vi "LUCS001RT_Navigation1_DataExchanger.vi"(7 "GPS DataIn":T1={"WayPointDataGood"=TRUE, "Waypoint:XTE"=0.01, "Waypoint:SteeringDirection"="L", "WayPoint:OriginID"="", "Waypoint:DestinationID"="", "DestinationWaypoint.Latitude.Deg"=0, "DestinationWaypoint.Latitude.Min"=0.0, "DestinationWaypointLatitude.North/South"="", "DestinationWaypointLongitude.Deg"=0, "DestinationWaypointLongitude.Min"=0.0, "DestinationWaypointLongitude.East/West"="", "RangeToDestination(NauticalMiles)"=0.0, "TrueBearingToDestination"=33.7, "VelocityTowardsDestination(Knots)"=0.0, "ArrivalAlarm"=TRUE, "ITOW"=247, "TAcc"=0, "LON"=0.0, "LAT"=0.0, "HEIGHT"=0, "HMSL"=0, "Hacc"=0, "Vacc"=0, "MSTOW"=0, "FixType"=0, "ECEF_X_Coor"=0, "ECEF_Y_Coor"=0, "ECEF_Z_Coor"=0, "Pacc"=0, "ECEF_X_Vlsty"=0, "ECEF_Y_Vlsty"=0, "ECEF_Z_Vlsty"=0, "Sacc"=0, "PosDOP"=0, "#SatsInNavSol"=0, "NED_NVsty"=0, "NED_Evsty"=0, "NED_DNvsty"=0, "Speed(3-D)"=0, "GSpeed(2-D)"=0, "Heading(2-D)"=0.0, "CAcc"=0, "Nano"=0, "Year"=0, "Month"=0, "Day"=0, "Hour"=0, "Min"=0, "Sec"=0, "UTC Valid"=0} {"UTC Valid" items=["UTC not valid", "Valid Time of Week", "Valid Week Number", "NA", "Valid UTC"]; "CAcc" format="%.0f°"; "Heading(2-D)" format="%0.6f°"; "GSpeed(2-D)" format="%.0f cm/s"; "Speed(3-D)" format="%.0f cm/s"; "NED_DNvsty" format="%.0f cm/s"; "NED_Evsty" format="%.0f cm/s"; "NED_NVsty" format="%.0f cm/s"; "Sacc" format="%.0f cm/s"; "ECEF_Z_Vlsty" format="%.0f cm/s"; "ECEF_Y_Vlsty" format="%.0f cm/s"; "ECEF_X_Vlsty" format="%.0f cm/s"; "FixType" items=["No Fix", "Dead Reckoning Only", "2D-Fix", "3D-Fix", "GPS + Dead Reckoning", "Time Only Fix", "RESERVED"]; "Vacc" format="%.0f mm"; "Hacc" format="%.0f mm"; "HMSL" format="%d mm"; "HEIGHT" format="%.0f mm"; "LAT" format="%#.6f"; "LON" format="%#.6f"; "Waypoint:XTE" format="%#.2f"}, 8 "error in (no error)":errorcluster, 11 "NavParam":T3={"Lat1Hem"=33.0, "Lat1Rad"=57.0, "Lon1Hem"=0.0, "Lon1Rad"=0.0, "Lat2Hem"=118.0, "Lat2Rad"=24.0, "Lon2Hem"=0.0, "Lon2Rad"=0.0, "DistanceRad"=40.0, "DistanceNM"=38.0, "CourseCond"=0.0, "TrueCourseRad"=0.0, "LatDegCurr"=73, "LatMinCurr"=47.0, "LatHemCurr"=0.0, "LatRadCurr"=0.0, "LonDegCurr"=0, "LonMinCurr"=0.0, "LonHemCurr"=0.0, "LonRadCurr"=-0.7023601432666094, "XTD"=40.0, "DistCurrRad"=38.0, "TrueCourseCurrRad"=0.0, "DistCurrNM"=0.7091854527270293, "TrueCourseDeg"=73.0, "TrueCourseCurrDeg"=47.0, "LON1"=0.0, "LAT1"=1.2877620997631494, "LON2"=38.0, "LAT2"=38.0} {"DistanceNM" format="%#.3f"}) -> (0 "error out":errorcluster, 3 "NavParamOut":T2={"Lat1Hem"=33.0, "Lat1Rad"=57.0, "Lon1Hem"=0.0, "Lon1Rad"=0.5925392810520749, "Lat2Hem"=118.0, "Lat2Rad"=24.0, "Lon2Hem"=0.0, "Lon2Rad"=2.066469834361286, "DistanceRad"=40.0, "DistanceNM"=38.0, "CourseCond"=0.0, "TrueCourseRad"=0.7091854527270293, "LatDegCurr"=73, "LatMinCurr"=47.0, "LatHemCurr"=0.0, "LatRadCurr"=1.2877620997631494, "LonDegCurr"=1, "LonMinCurr"=2143.726101388629, "LonHemCurr"=-0.7023601432666094, "LonRadCurr"=-0.7023601432666094, "XTD"=40.0, "DistCurrRad"=38.0, "TrueCourseCurrRad"=0.0, "DistCurrNM"=0.7091854527270293, "TrueCourseDeg"=73.0, "TrueCourseCurrDeg"=47.0, "LON1"=0.0, "LAT1"=1.2877620997631494, "LON2"=38.0, "LAT2"=38.0} {"DistanceNM" format="%#.3f"})   [LabVIEW 2020]
uses:
  TypeDefs/NavigationParams.ctl
  LUCS001RT_GPS_Data.ctl
  GPS_Navigation_Parameters.ctl
panel:
  # "WAYPOINT"
  # "CURRENT POSITION"
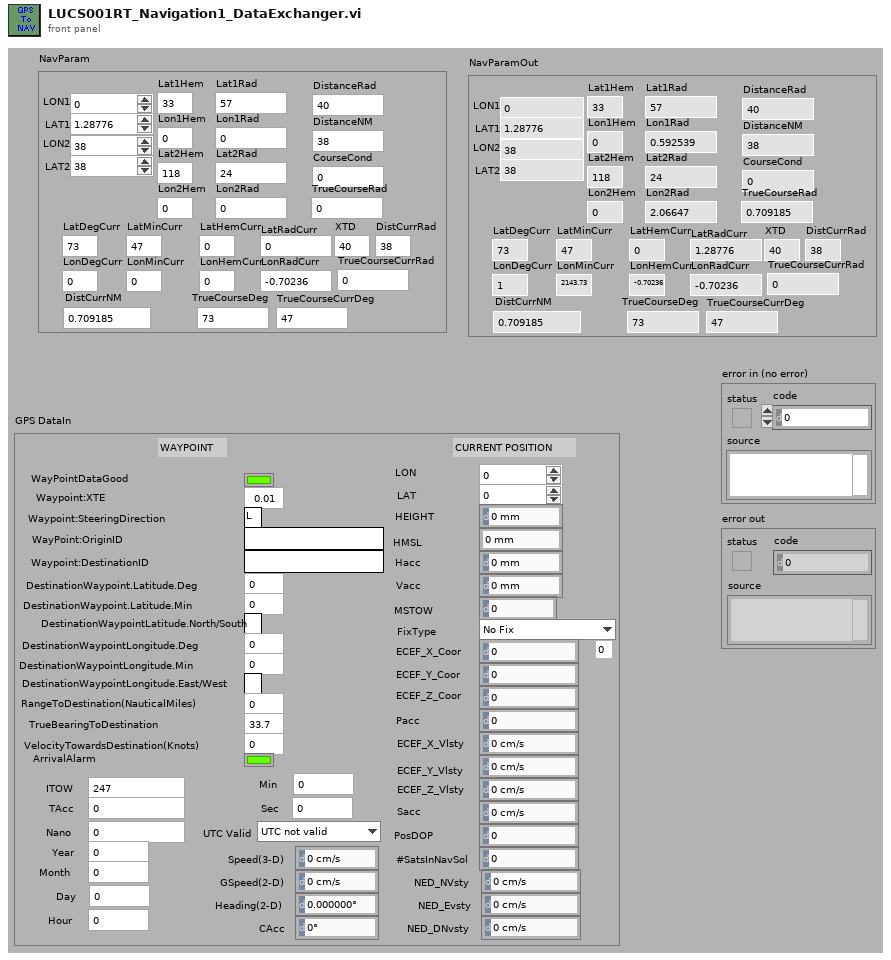
[diagram p1: front panel]
types:
  T1 = typedef "LUCS001RT_GPS_Data.ctl" = cluster{"WayPointDataGood":bool, "Waypoint:XTE":dbl, "Waypoint:SteeringDirection":string, "WayPoint:OriginID":string, "Waypoint:DestinationID":string, "DestinationWaypoint.Latitude.Deg":i32, "DestinationWaypoint.Latitude.Min":dbl, "DestinationWaypointLatitude.North/South":string, "DestinationWaypointLongitude.Deg":i32, "DestinationWaypointLongitude.Min":dbl, "DestinationWaypointLongitude.East/West":string, "RangeToDestination(NauticalMiles)":dbl, "TrueBearingToDestination":dbl, "VelocityTowardsDestination(Knots)":dbl, "ArrivalAlarm":bool, "ITOW":u32, "TAcc":u32, "LON":dbl, "LAT":dbl, "HEIGHT":i32, "HMSL":i32, "Hacc":u32, "Vacc":u32, "MSTOW":u32, "FixType":u8, "ECEF_X_Coor":i32, "ECEF_Y_Coor":i32, "ECEF_Z_Coor":i32, "Pacc":u32, "ECEF_X_Vlsty":i32, "ECEF_Y_Vlsty":i32, "ECEF_Z_Vlsty":i32, "Sacc":u32, "PosDOP":u16, "#SatsInNavSol":u8, "NED_NVsty":i32, "NED_Evsty":i32, "NED_DNvsty":i32, "Speed(3-D)":u32, "GSpeed(2-D)":u32, "Heading(2-D)":dbl, "CAcc":u32, "Nano":i32, "Year":u16, "Month":u8, "Day":u8, "Hour":u8, "Min":u8, "Sec":u8, "UTC Valid":u8}
  T2 = typedef "NavigationParams.ctl" = cluster{"Lat1Hem":dbl, "Lat1Rad":dbl, "Lon1Hem":dbl, "Lon1Rad":dbl, "Lat2Hem":dbl, "Lat2Rad":dbl, "Lon2Hem":dbl, "Lon2Rad":dbl, "DistanceRad":dbl, "DistanceNM":dbl, "CourseCond":dbl, "TrueCourseRad":dbl, "LatDegCurr":i32, "LatMinCurr":dbl, "LatHemCurr":dbl, "LatRadCurr":dbl, "LonDegCurr":i32, "LonMinCurr":dbl, "LonHemCurr":dbl, "LonRadCurr":dbl, "XTD":dbl, "DistCurrRad":dbl, "TrueCourseCurrRad":dbl, "DistCurrNM":dbl, "TrueCourseDeg":dbl, "TrueCourseCurrDeg":dbl, "LON1":dbl, "LAT1":dbl, "LON2":dbl, "LAT2":dbl}
  T3 = typedef "GPS_Navigation_Parameters.ctl" = cluster{"Lat1Hem":dbl, "Lat1Rad":dbl, "Lon1Hem":dbl, "Lon1Rad":dbl, "Lat2Hem":dbl, "Lat2Rad":dbl, "Lon2Hem":dbl, "Lon2Rad":dbl, "DistanceRad":dbl, "DistanceNM":dbl, "CourseCond":dbl, "TrueCourseRad":dbl, "LatDegCurr":i32, "LatMinCurr":dbl, "LatHemCurr":dbl, "LatRadCurr":dbl, "LonDegCurr":i32, "LonMinCurr":dbl, "LonHemCurr":dbl, "LonRadCurr":dbl, "XTD":dbl, "DistCurrRad":dbl, "TrueCourseCurrRad":dbl, "DistCurrNM":dbl, "TrueCourseDeg":dbl, "TrueCourseCurrDeg":dbl, "LON1":dbl, "LAT1":dbl, "LON2":dbl, "LAT2":dbl}
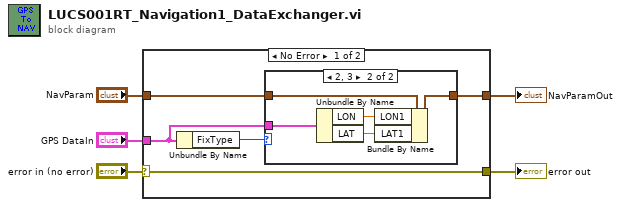
[diagram p0: block diagram]
diagram:
  n1 = case shown="No Error" "error in (no error)" {
    selector: "error in (no error)" -> [w10 w17]
    tunnel: "NavParam" -> [w7 _]
    tunnel: [w10 w17] -> w3
    tunnel: "GPS DataIn" -> [w8 _]
    tunnel: [w6 _] -> w1
    frame No Error {
      n2 = Unbundle By Name(w8) -> ("FixType"=w9:u8)
      n3 = case shown="2, 3" w9 {
        tunnel: w8 -> [_ w16]
        tunnel: w7 -> [w11 w15]
        tunnel: [w11 w12] -> w6
        frame 0, Default {
        }
        frame 2, 3 {
          n4 = Unbundle By Name(w16) -> ("LON"=w14:dbl, "LAT"=w13:dbl)
          n5 = Bundle By Name(cluster=w15, "LON1"=w14, "LAT1"=w13) -> (w12:T3)
        }
      }
    }
    frame Error {
    }
  }
  "NavParamOut" <- w1
  "error out" <- w3
